vi "GUI_passive_Somatic_Test.vi"(0 "lang":string, 2 "Do test?":bool, 3 "Total trial":u16=80 min=1, 4 "Direction":i8=45) -> (7 "Direction 2":i8=20, 8 "stop 2":bool)   [LabVIEW 2012]
uses:
  <vilib>/Analysis/NI_AALBase.lvlib
  subVIs/Global_var.vi
  <vilib>/Utility/file.llb/Write To Spreadsheet File (DBL).vi
  <vilib>/Analysis/1siggen.llb/Riffle Array (I32).vi
panel:
  out "Response":u8
  out "Test Type":string
  out "Trial_index":u16
  out "Correct?":bool
  out "Response":path
  out "Trajectory":path
  out "Current Seq":u8
  out "Target":dbl[](array[numeric])
  out "flag":bool
  out "Directions":dbl[](array[numeric])
  out "Fz":dbl
  out "X":dbl
  out "Y":dbl
  out "Z":dbl
  out "Vx":dbl
  out "Vy":dbl
  out "Vz":dbl
  out "error out":errorcluster
  in  "Start?":bool
  out "Fx":dbl
  out "Fy":dbl
  out "Trial #":u16
  in  "stop":bool
  out "Canvas":picture
  # "Is the movement to the right or left of the body midline?"
  # "Delta robot kinetics information"
  # "degree"
types:
  T1 = typedef "Sound Output Task ID.ctl" = u32
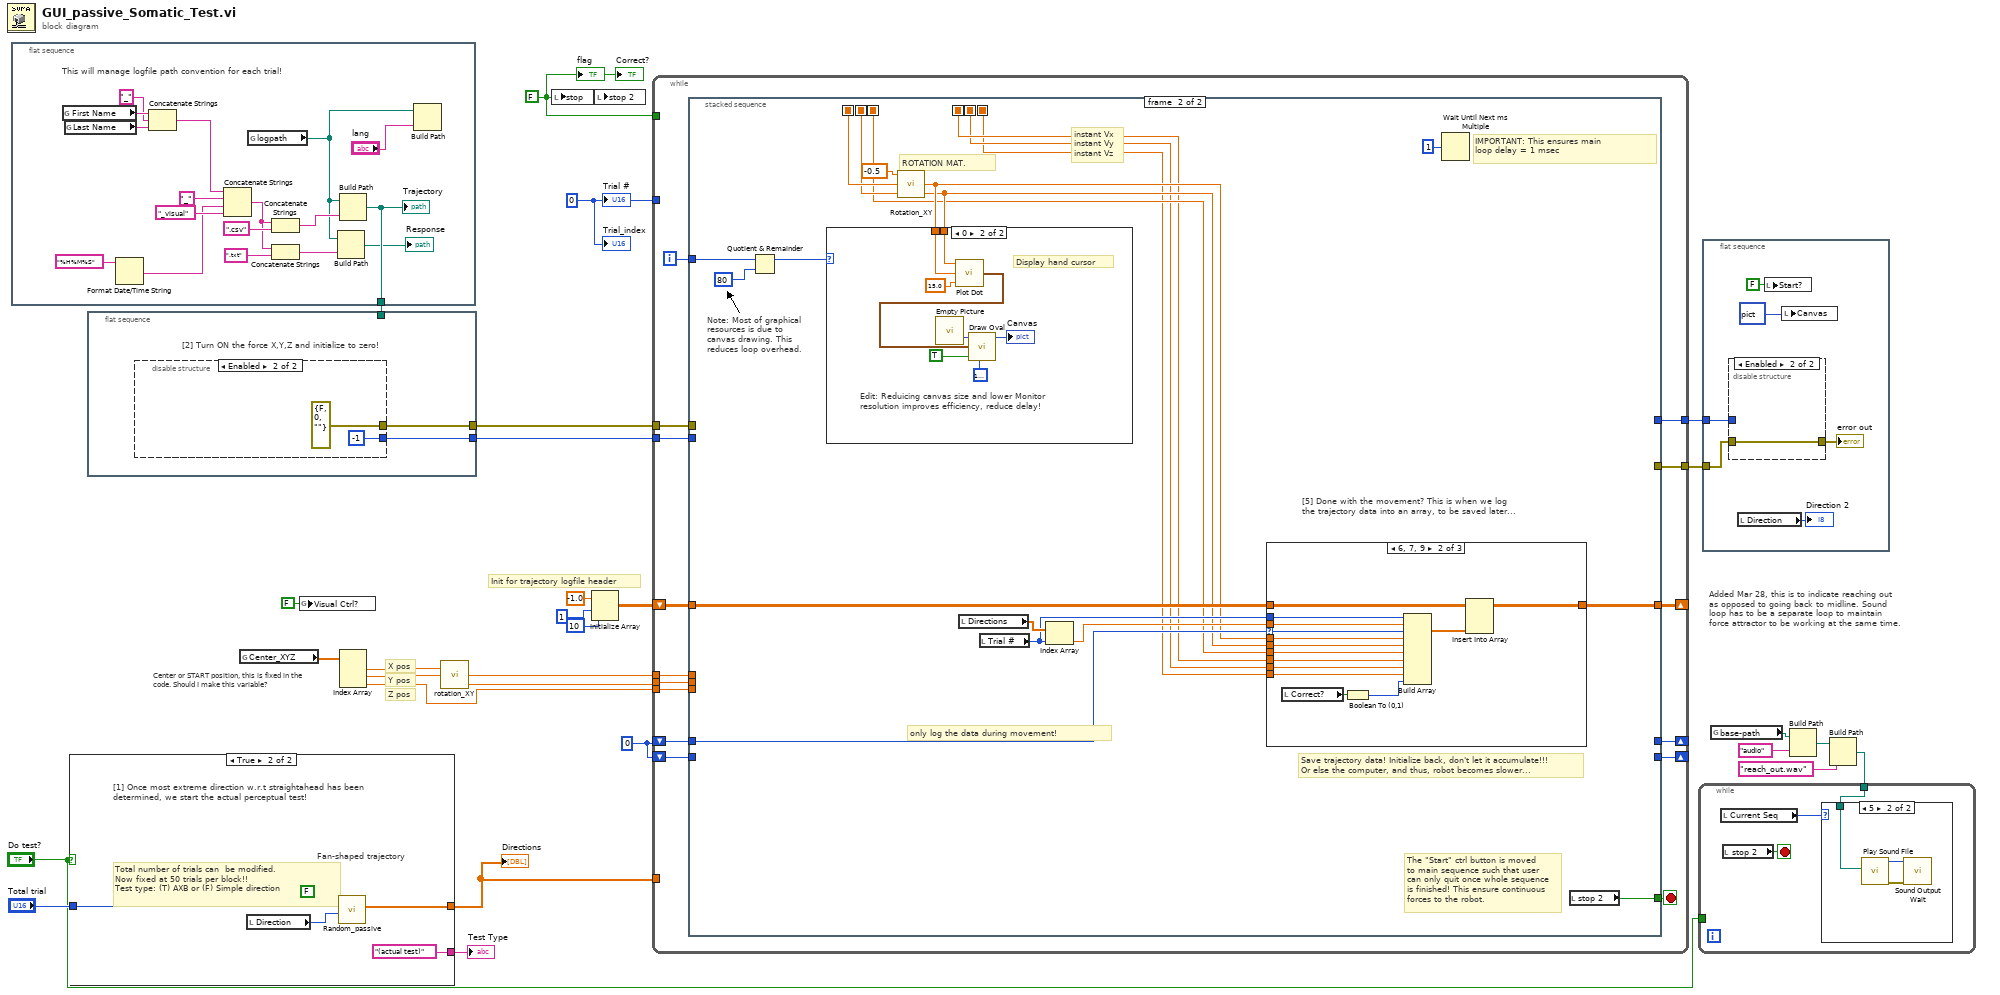
[diagram p0: block diagram]
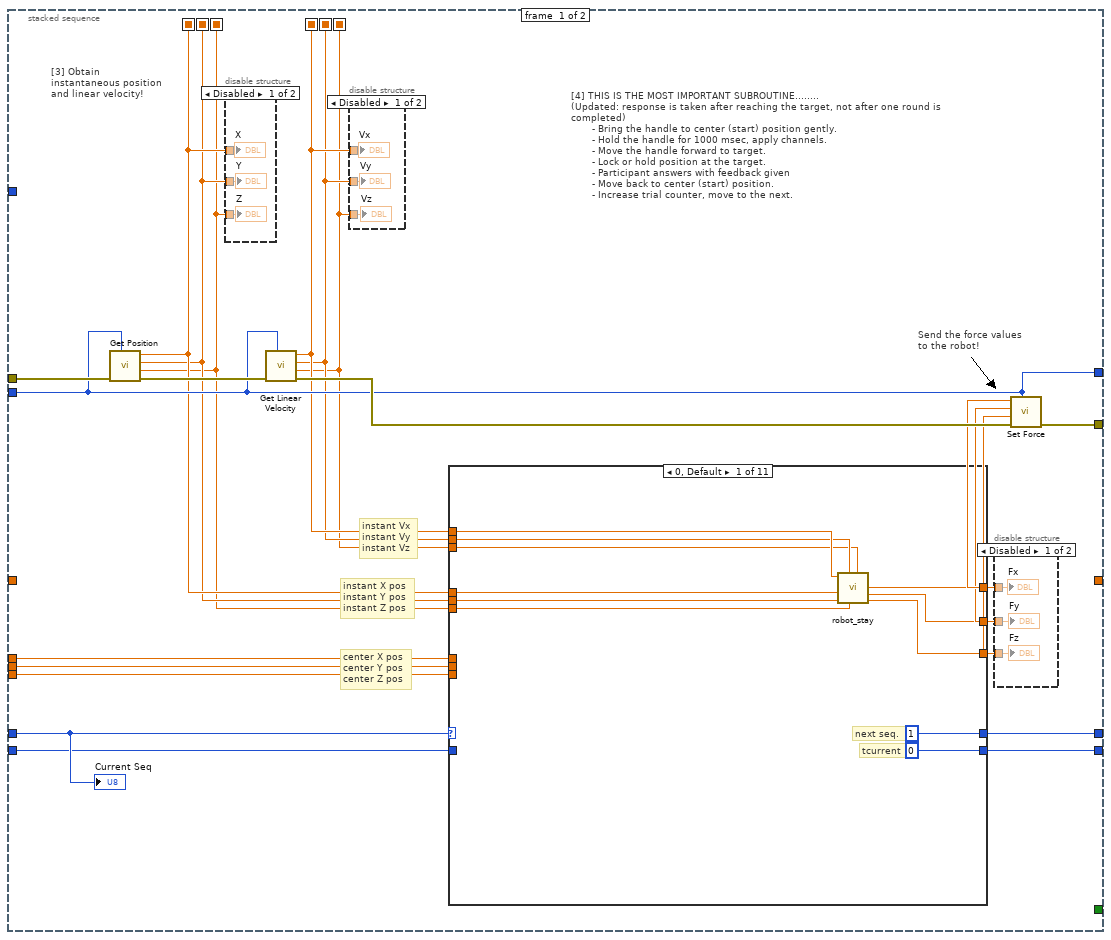
[diagram p3: hidden frame]
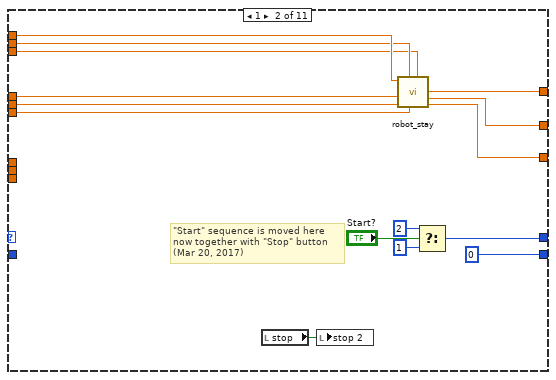
[diagram p7: hidden frame]
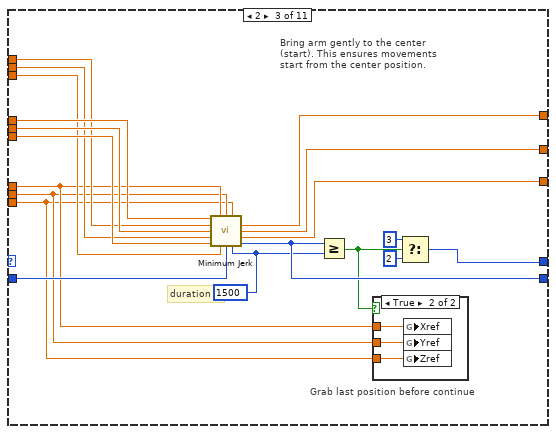
[diagram p8: hidden frame]
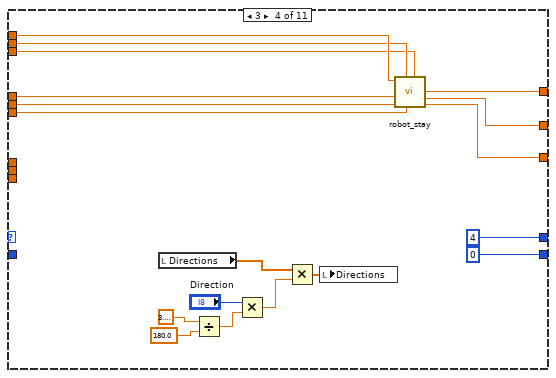
[diagram p10: hidden frame]
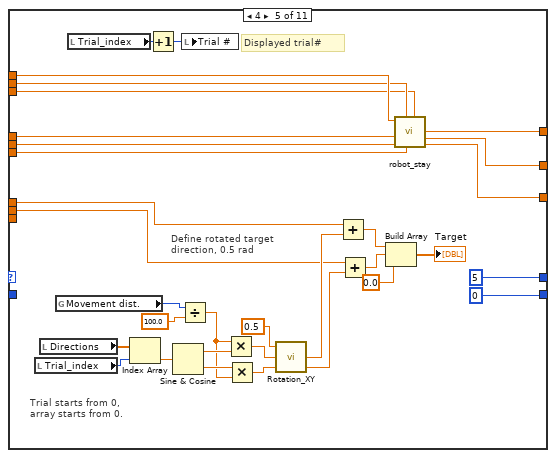
[diagram p11: hidden frame]
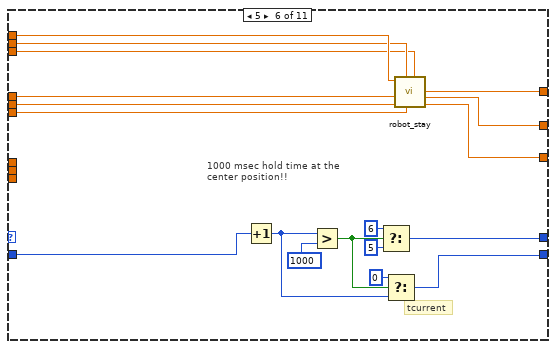
[diagram p12: hidden frame]
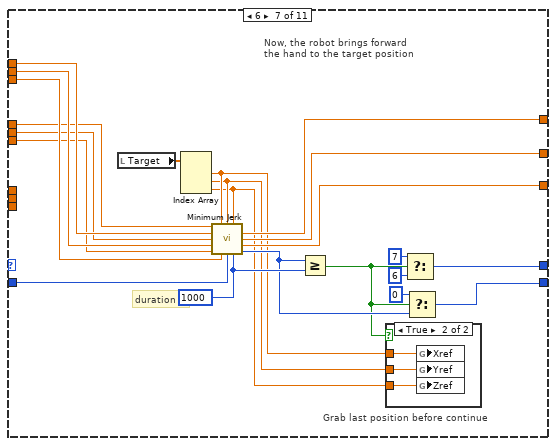
[diagram p13: hidden frame]
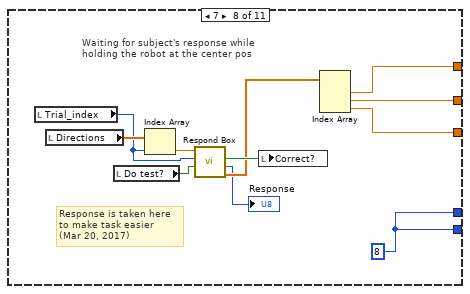
[diagram p15: hidden frame]
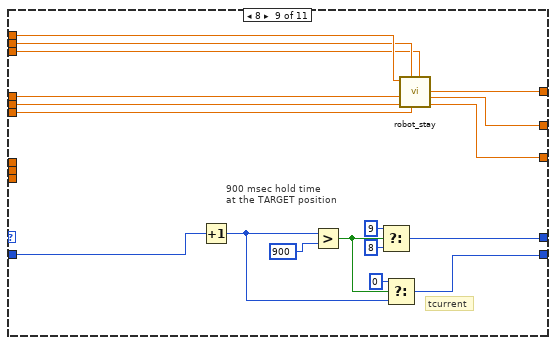
[diagram p16: hidden frame]
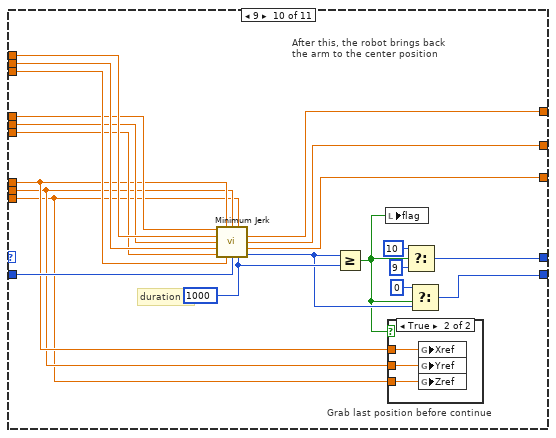
[diagram p17: hidden frame]
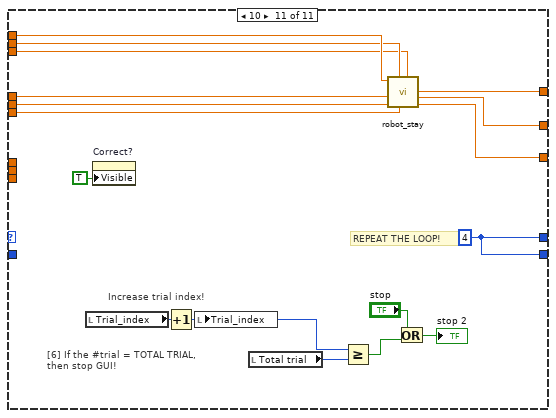
[diagram p19: hidden frame]
diagram:
  w16 = u16 0 ("y")
  w23 = FALSE ("stop")
  w25 = u16 0 ("ID")
  # "Added Mar 28, this is to indicate reaching out\nas opposed to going back to midline. Sound\nloop has to be a separate loop to maintain\nforce attractor to be working at the same time."
  # "Z pos"
  # "Y pos"
  # "X pos"
  # "Center or START position, this is fixed in the code. Should I make this variable?"
  # "Init for trajectory logfile header"
  n1 = flat-sequence {
    tunnel: [w31] -> w1
    frame #0 {
      # "This will manage logfile path convention for each trial!"
      n2 = global read "Global_var.vi" "First Name"() -> (w41:string)
      n3 = global read "Global_var.vi" "Last Name"() -> (w39:string)
      n4 = Format Date/Time String(time format string (%c)="%H%M%S") -> (date/time string=w43:string)  [unwired: 2 in]
      n5 = Concatenate Strings(w41, "_" ("string"), w39) -> (w38:string)
      n6 = Concatenate Strings(w38, "_" ("string"), w43, "_visual" ("string")) -> (w36:string)
      n7 = global read "Global_var.vi" "logpath"() -> (w33:path)
      n8 = Concatenate Strings(w36, ".csv" ("string")) -> (w34:string)
      n9 = Concatenate Strings(w36, ".txt" ("string")) -> (w32:string)
      n10 = Build Path(base path=w33, name or relative path=w32) -> (appended path=→"Response":path)
      n11 = Build Path(base path=w33, name or relative path=w34) -> (appended path=w31:path)
      "Trajectory" <- w31
      n12 = Build Path(base path=w33, name or relative path="lang") -> ()  [unwired: 1 out]
    }
  }
  n13 = case shown="True" "Do test?" {
    tunnel: [w46 w61] -> w12
    tunnel: "Total trial" -> [_ w60]
    tunnel: ["(extreme test) " "(actual test)"] -> w17
    frame False {
      # "[1] Determine min. perceivable direction, and randomise the presentation. (Darainy, 2017)."
      # "shuffle"
      n14 = local read "Total trial"() -> (w56:u16)
      n15 = Divide(x=w56, y=u8 2) -> (x/y=w55:dbl)
      n16 = Divide(x=w56, y=u8 2) -> (x/y=w50:dbl)
      n17 = Initialize Array(i8 1 ("element"), w55) -> (w49:i8[])
      n18 = Initialize Array(i8 -1 ("element"), w50) -> (w48:i8[])
      n19 = Build Array (concatenate)(w49, w48) -> (w47:i8[])
      n20 = call-poly <vilib>:"Riffle.vi"("X"=w47) -> ("Riffled {X}"=w46:i32[])  [unwired: 8 in, 2 out]
    }
    frame True {
      # "Fan-shaped trajectory"
      # "Total number of trials can  be modified.\nNow fixed at 50 trials per block!!\nTest type: (T) AXB or (F) Simple direction"
      # "[1] Once most extreme direction w.r.t straightahead has been determined, we start the actual perceptual test!"
      n21 = local read "Direction"() -> (w62:i8)
      n22 = call "Random_passive.vi"("Degree Max."=w62, "Total trial"=w60, "Test mode\n(Simple or AXB paradigm)?"=FALSE ("Test mode\n(Simple or AXB paradigm)?")) -> ("Target"=w61:dbl[])  [unwired: 5 in, 3 out]
    }
  }
  "Test Type" <- w17
  "Directions" <- w12
  n23 = flat-sequence {
    tunnel: [w64] -> w27
    tunnel: [w63] -> w26
    tunnel: w1 -> [_]
    frame #0 {
      # "[2] Turn ON the force X,Y,Z and initialize to zero!"
      n24 = disable-structure shown="Enabled" {
        disable-tunnel: [w66 errorcluster {"status"=FALSE, "code"=0, "source"=""} ("error out")] -> w64
        disable-tunnel: [w65 i8 -1 ("ID")] -> w63
        frame Disabled {
          w65 = i8 -1 ("ID")
          n25 = call <userlib>:"Open.vi"("error in (no error)"=errorcluster {"status"=FALSE, "code"=0, "source"=""} ("error out")) -> ("error out"=w67:errorcluster)  [unwired: 9 in, 1 out]
          n26 = call <userlib>:"Enable Force.vi"("error in (no error)"=w67, "ID"=w65, "val"=u8 1) -> ("error out"=w66:errorcluster)  [unwired: 7 in, 1 out]
        }
        frame Enabled {
        }
      }
    }
  }
  n27 = global read "Global_var.vi" "Center_XYZ"() -> (w13:dbl[])
  n28 = global write "Global_var.vi" "Visual Ctrl?"(FALSE ("Visual Ctrl?")) -> ()
  n29 = Index Array(array=w13) -> (element #1=w15:dbl, element #2=w14:dbl, element #3=w11:dbl)  [unwired: 3 in]
  n30 = call "rotation_XY.vi"("x_pos"=w14, "angle"=w15) -> ("rot_y"=w10:dbl, "rot_x"=w9:dbl)  [unwired: 2 in]
  n31 = local write "stop"(w23) -> ()
  n32 = Initialize Array(-1.0 ("vz out"), 1 ("dimension size"), 10 ("dimension size")) -> (w22:dbl[][])
  n33 = local write "stop 2"(w23) -> ()
  n34 = while {
    tunnel: w26 -> [w85]
    shift-right: [w86] -> _
    shift-left: w25 -> [w81]
    shift-right: [w83] -> _
    shift-left: w22 -> [w82]
    tunnel: [w79] -> w28
    tunnel: w16 -> [_]
    tunnel: w27 -> [w78]
    shift-right: [w76] -> _
    shift-left: w25 -> [w77]
    tunnel: w23 -> [_]
    tunnel: [w75] -> w24
    tunnel: w12 -> [_]
    tunnel: w9 -> [w74]
    tunnel: w10 -> [w73]
    tunnel: w11 -> [w72]
    i -> [w80]
    stop <- w84 stop-if-true
    n35 = stacked-sequence {
      seq-local: [w93 _] -> [_ w332]
      seq-local: [w90 _] -> [_ w329]
      seq-local: [w92 _] -> [_ w331]
      seq-local: [w91 _] -> [_ w330]
      seq-local: [w94 _] -> [_ w335]
      seq-local: [w95 _] -> [_ w336]
      tunnel: [w106 _] -> w86
      tunnel: w85 -> [w99 _]
      tunnel: [_ w328] -> w84
      tunnel: [_ w342] -> w83
      tunnel: w82 -> [_ w341]
      tunnel: w81 -> [w107 w338]
      tunnel: w80 -> [_ w346]
      tunnel: [w99 _] -> w79
      tunnel: w78 -> [w101 _]
      tunnel: w77 -> [w105 _]
      tunnel: [w104 _] -> w76
      tunnel: [w103 _] -> w75
      tunnel: w74 -> [w89 _]
      tunnel: w73 -> [w88 _]
      tunnel: w72 -> [w87 _]
      frame #0 {
        # "center X pos\ncenter Y pos\ncenter Z pos"
        # "[3] Obtain instantaneous position and linear velocity!"
        # "Send the force values to the robot!"
        # "instant Vx\ninstant Vy\ninstant Vz"
        # "[4] THIS IS THE MOST IMPORTANT SUBROUTINE........\n(Updated: response is taken after reaching the target, not after one round is completed)\n       - Bring the handle to center (start) position gently.\n       - Hold the handle for 1000 msec, apply channels.\n       - Move the handle forward to target.\n       - Lock or hold position at the target.\n       - Participant answers with feedback given\n       - Move back to center (start) position.\n       - Increase trial counter, move to the next."
        # "instant X pos\ninstant Y pos\ninstant Z pos"
        n36 = call <userlib>:"Get Position.vi"("ID"=w99, "error in (no error)"=w101) -> ("error out"=w102:errorcluster, "pz out"=w93:dbl, "py out"=w94:dbl, "px out"=w95:dbl)  [unwired: 5 in, 1 out]
        n37 = disable-structure shown="Disabled" {
          disable-tunnel: w95 -> [w113 _]
          disable-tunnel: w94 -> [w112 _]
          disable-tunnel: w93 -> [w111 _]
          frame Disabled {
            "Z" <- w111
            "Y" <- w112
            "X" <- w113
          }
          frame Enabled {
          }
        }
        n38 = call <userlib>:"Get Linear Velocity.vi"("ID"=w99, "error in (no error)"=w102) -> ("error out"=w100:errorcluster, "vz out"=w90:dbl, "vy out"=w91:dbl, "vx out"=w92:dbl)  [unwired: 5 in, 1 out]
        n39 = disable-structure shown="Disabled" {
          disable-tunnel: w92 -> [w116 _]
          disable-tunnel: w91 -> [w115 _]
          disable-tunnel: w90 -> [w114 _]
          frame Disabled {
            "Vz" <- w114
            "Vy" <- w115
            "Vx" <- w116
          }
          frame Enabled {
          }
        }
        n40 = case shown="0, Default" w107 {
          tunnel: [u8 1 ("ID") w128 w159 u8 4 ("ID") u8 5 ("ID") w232 w241 w268 w283 w294 w326] -> w106
          tunnel: [w122 w135 w155 w175 w185 w223 w244 w261 w271 w298 w322] -> w98
          tunnel: [w121 w134 w156 w174 w183 w222 w243 w263 w270 w297 w321] -> w97
          tunnel: w105 -> [_ _ w153 _ _ w230 w245 _ w279 w295 _]
          tunnel: [u16 0 ("tcurrent") u32 0 ("millisecond timer value") w158 u32 0 ("ID") u32 0 ("ID") w231 w239 w268 w281 w291 w326] -> w104
          tunnel: [w120 w133 w157 w173 w184 w221 w242 w262 w269 w296 w320] -> w96
          tunnel: w95 -> [w119 w138 w152 w178 w188 w226 w248 _ w274 w301 w325]
          tunnel: w94 -> [w118 w137 w151 w177 w187 w225 w247 _ w273 w300 w324]
          tunnel: w93 -> [w117 w136 w150 w176 w186 w224 w246 _ w272 w299 w323]
          tunnel: w92 -> [w125 w141 w149 w181 w191 w229 w251 _ w277 w304 w319]
          tunnel: w91 -> [w124 w140 w148 w180 w190 w228 w250 _ w276 w303 w318]
          tunnel: w90 -> [w123 w139 w147 w179 w189 w227 w249 _ w275 w302 w317]
          tunnel: w89 -> [_ _ w145 _ w197 _ _ _ _ w289 _]
          tunnel: w88 -> [_ _ w144 _ w196 _ _ _ _ w288 _]
          tunnel: w87 -> [_ _ w143 _ _ _ _ _ _ w287 _]
          frame 0, Default {
            # "next seq."
            # "tcurrent"
            n41 = call "robot_stay.vi"("Vz"=w123, "Z"=w117, "Vy"=w124, "Y"=w118, "X"=w119, "Vx"=w125) -> ("Fz"=w120:dbl, "Fy"=w121:dbl, "Fx"=w122:dbl)  [unwired: 3 in]
          }
          frame 1 {
            # "\"Start\" sequence is moved here \nnow together with \"Stop\" button\n(Mar 20, 2017)"
            n42 = local read "stop"() -> (w129:bool)
            n43 = local write "stop 2"(w129) -> ()
            n44 = call "robot_stay.vi"("Vz"=w139, "Z"=w136, "Vy"=w140, "Y"=w137, "X"=w138, "Vx"=w141) -> ("Fz"=w133:dbl, "Fy"=w134:dbl, "Fx"=w135:dbl)  [unwired: 3 in]
            n45 = Select(t=u8 2, s="Start?", f=u8 1) -> (s? t:f=w128:u8)
          }
          frame 2 {
            w154 = u16 1500 ("duration")
            # "Grab last position before continue"
            # "Bring arm gently to the center\n(start). This ensures movements\nstart from the center position."
            # "duration"
            n46 = call "Minimum Jerk.vi"("X"=w152, "Xfinal"=w145, "Yfinal"=w144, "Zfinal"=w143, "Vx"=w149, "Y"=w151, "Vy"=w148, "Z"=w150, "Vz"=w147, "current_n"=w153, "duration"=w154) -> ("Fx"=w155:dbl, "Fy"=w156:dbl, "Fz"=w157:dbl, "n out"=w158:u16)  [unwired: 1 out]
            n47 = Greater Or Equal?(x=w158, y=w154) -> (x >= y?=w146:bool)
            n48 = case shown="True" w146 {
              tunnel: w145 -> [_ w164]
              tunnel: w144 -> [_ w163]
              tunnel: w143 -> [_ w162]
              frame False {
              }
              frame True {
                n49 = global write "Global_var.vi" "Xref"(w164) -> ()
                n50 = global write "Global_var.vi" "Yref"(w163) -> ()
                n51 = global write "Global_var.vi" "Zref"(w162) -> ()
              }
            }
            n52 = Select(t=u8 3 ("ID"), s=w146, f=u8 2) -> (s? t:f=w159:u8)
          }
          frame 3 {
            n53 = local read "Directions"() -> (w166:dbl[])
            n54 = Divide(x=3.141592653589793, y=180.0) -> (x/y=w169:dbl)
            n55 = Multiply(x="Direction", y=w169) -> (x*y=w172:dbl)
            n56 = Multiply(x=w166, y=w172) -> (x*y=w167:dbl[])
            n57 = local write "Directions"(w167) -> ()
            n58 = call "robot_stay.vi"("Vz"=w179, "Z"=w176, "Vy"=w180, "Y"=w177, "X"=w178, "Vx"=w181) -> ("Fz"=w173:dbl, "Fy"=w174:dbl, "Fx"=w175:dbl)  [unwired: 3 in]
          }
          frame 4 {
            # "Displayed trial#"
            # "Trial starts from 0,\narray starts from 0."
            # "Define rotated target direction, 0.5 rad"
            n59 = local read "Trial_index"() -> (w210:u16)
            n60 = local read "Directions"() -> (w211:dbl[])
            n61 = global read "Global_var.vi" "Movement dist."() -> (w209:u8)
            n62 = local read "Trial_index"() -> (w192:u16)
            n63 = Index Array(array=w211, index=w210) -> (element=w212:dbl)
            n64 = Increment(x=w192) -> (x+1=w193:u16)
            n65 = Sine & Cosine(0:w212) -> (1:w213:dbl, 2:w214:dbl)
            n66 = Divide(x=w209, y=100.0) -> (x/y=w207:dbl)
            n67 = local write "Trial #"(w193) -> ()
            n68 = Multiply(x=w207, y=w213) -> (x*y=w205:dbl)
            n69 = Multiply(x=w214, y=w207) -> (x*y=w206:dbl)
            n70 = call "Rotation_XY.vi"("y_pos"=w206, "x_pos"=w205, "angle"=0.5 ("theta")) -> ("rot_y"=w202:dbl, "rot_x"=w203:dbl)  [unwired: 1 in]
            n71 = Add(x=w197, y=w203) -> (x+y=w200:dbl)
            n72 = Add(x=w196, y=w202) -> (x+y=w199:dbl)
            n73 = Build Array(w200, w199, 0.0 ("element")) -> (→"Target":dbl[])
            n74 = call "robot_stay.vi"("Vz"=w189, "Z"=w186, "Vy"=w190, "Y"=w187, "X"=w188, "Vx"=w191) -> ("Fz"=w184:dbl, "Fy"=w183:dbl, "Fx"=w185:dbl)  [unwired: 3 in]
          }
          frame 5 {
            # "1000 msec hold time at the center position!!"
            # "tcurrent"
            n75 = Increment(x=w230) -> (x+1=w215:u32)
            n76 = Greater?(x=w215, y=u32 1000) -> (0:w216:bool)
            n77 = Select(t=u8 6 ("ID"), s=w216, f=u8 5) -> (s? t:f=w232:u8)
            n78 = Select(t=u8 0 ("ID"), s=w216, f=w215) -> (s? t:f=w231:u32)
            n79 = call "robot_stay.vi"("Vz"=w227, "Z"=w224, "Vy"=w228, "Y"=w225, "X"=w226, "Vx"=w229) -> ("Fz"=w221:dbl, "Fy"=w222:dbl, "Fx"=w223:dbl)  [unwired: 3 in]
          }
          frame 6 {
            w252 = u16 1000 ("duration")
            # "Grab last position before continue"
            # "Now, the robot brings forward\nthe hand to the target position"
            # "duration"
            n80 = local read "Target"() -> (w237:dbl[])
            n81 = Index Array(array=w237) -> (element #1=w235:dbl, element #2=w234:dbl, element #3=w233:dbl)  [unwired: 3 in]
            n82 = call "Minimum Jerk.vi"("X"=w248, "Xfinal"=w235, "Yfinal"=w234, "Zfinal"=w233, "Vx"=w251, "Y"=w247, "Vy"=w250, "Z"=w246, "Vz"=w249, "current_n"=w245, "duration"=w252) -> ("Fx"=w244:dbl, "Fy"=w243:dbl, "Fz"=w242:dbl, "n out"=w238:u16)  [unwired: 1 out]
            n83 = Greater Or Equal?(x=w238, y=w252) -> (x >= y?=w236:bool)
            n84 = case shown="True" w236 {
              tunnel: w235 -> [_ w257]
              tunnel: w234 -> [_ w256]
              tunnel: w233 -> [_ w255]
              frame False {
              }
              frame True {
                n85 = global write "Global_var.vi" "Xref"(w257) -> ()
                n86 = global write "Global_var.vi" "Yref"(w256) -> ()
                n87 = global write "Global_var.vi" "Zref"(w255) -> ()
              }
            }
            n88 = Select(t=u8 7 ("ID"), s=w236, f=u8 6) -> (s? t:f=w241:u8)
            n89 = Select(t=u16 0, s=w236, f=w238) -> (s? t:f=w239:u16)
          }
          frame 7 {
            w268 = u8 8 ("ID")
            # "Response is taken here\nto make task easier\n(Mar 20, 2017)"
            # "Waiting for subject's response while\nholding the robot at the center pos"
            n90 = local read "Trial_index"() -> (w259:u16)
            n91 = local read "Directions"() -> (w267:dbl[])
            n92 = local read "Do test?"() -> (w260:bool)
            n93 = Index Array(array=w267, index=w259) -> (element=w266:dbl)
            n94 = call "Respond Box.vi"("Play?"=w260, "Trial#"=w259, "target"=w266) -> ("Force"=w264:dbl[], "out"=→"Response":i8, "Correct?"=w265:bool)  [unwired: 3 in]
            n95 = local write "Correct?"(w265) -> ()
            n96 = Index Array(array=w264) -> (element #1=w261:dbl, element #2=w263:dbl, element #3=w262:dbl)  [unwired: 3 in]
          }
          frame 8 {
            # "900 msec hold time\nat the TARGET position"
            # "tcurrent"
            n97 = Increment(x=w279) -> (x+1=w278:u32)
            n98 = Greater?(x=w278, y=u32 900) -> (0:w280:bool)
            n99 = Select(t=u8 9 ("ID"), s=w280, f=u8 8) -> (s? t:f=w283:u8)
            n100 = Select(t=u8 0 ("ID"), s=w280, f=w278) -> (s? t:f=w281:u32)
            n101 = call "robot_stay.vi"("Vz"=w275, "Z"=w272, "Vy"=w276, "Y"=w273, "X"=w274, "Vx"=w277) -> ("Fz"=w269:dbl, "Fy"=w270:dbl, "Fx"=w271:dbl)  [unwired: 3 in]
          }
          frame 9 {
            w305 = u16 1000 ("duration")
            # "Grab last position before continue"
            # "After this, the robot brings back\nthe arm to the center position"
            # "duration"
            n102 = call "Minimum Jerk.vi"("X"=w301, "Xfinal"=w289, "Yfinal"=w288, "Zfinal"=w287, "Vx"=w304, "Y"=w300, "Vy"=w303, "Z"=w299, "Vz"=w302, "current_n"=w295, "duration"=w305) -> ("Fx"=w298:dbl, "Fy"=w297:dbl, "Fz"=w296:dbl, "n out"=w292:u16)  [unwired: 1 out]
            n103 = Greater Or Equal?(x=w292, y=w305) -> (x >= y?=w290:bool)
            n104 = local write "flag"(w290) -> ()
            n105 = case shown="True" w290 {
              tunnel: w289 -> [_ w310]
              tunnel: w288 -> [_ w309]
              tunnel: w287 -> [_ w308]
              frame False {
              }
              frame True {
                n106 = global write "Global_var.vi" "Xref"(w310) -> ()
                n107 = global write "Global_var.vi" "Yref"(w309) -> ()
                n108 = global write "Global_var.vi" "Zref"(w308) -> ()
              }
            }
            n109 = Select(t=u8 10 ("ID"), s=w290, f=u8 9) -> (s? t:f=w294:u8)
            n110 = Select(t=u16 0, s=w290, f=w292) -> (s? t:f=w291:u16)
          }
          frame 10 {
            w326 = u8 4 ("ID")
            # "REPEAT THE LOOP!"
            # "[6] If the #trial = TOTAL TRIAL, \nthen stop GUI!"
            # "Increase trial index!"
            n111 = local read "Trial_index"() -> (w316:u16)
            n112 = property on="Correct?" class="Bool (strict)"("Visible"=TRUE ("stop")) -> ()  [unwired: 2 in, 2 out]
            n113 = Increment(x=w316) -> (x+1=w314:u16)
            n114 = local write "Trial_index"(w314) -> ()
            n115 = local read "Total trial"() -> (w315:u16)
            n116 = Greater Or Equal?(x=w314, y=w315) -> (x >= y?=w311:bool)
            n117 = call "robot_stay.vi"("Vz"=w317, "Z"=w323, "Vy"=w318, "Y"=w324, "X"=w325, "Vx"=w319) -> ("Fz"=w320:dbl, "Fy"=w321:dbl, "Fx"=w322:dbl)  [unwired: 3 in]
            n118 = Or(x="stop", y=w311) -> (x .or. y?=→"stop 2":bool)
          }
        }
        n119 = disable-structure shown="Disabled" {
          disable-tunnel: w98 -> [w110 _]
          disable-tunnel: w97 -> [w109 _]
          disable-tunnel: w96 -> [w108 _]
          frame Disabled {
            "Fy" <- w109
            "Fx" <- w110
            "Fz" <- w108
          }
          frame Enabled {
          }
        }
        n120 = call <userlib>:"Set Force.vi"("ID"=w99, "error in (no error)"=w100, "fz"=w96, "fy"=w97, "fx"=w98) -> ("error out"=w103:errorcluster)  [unwired: 5 in, 1 out]
        "Current Seq" <- w107
      }
      frame #1 {
        # "Save trajectory data! Initialize back, don't let it accumulate!!!\nOr else the computer, and thus, robot becomes slower..."
        # "The \"Start\" ctrl button is moved\nto main sequence such that user\ncan only quit once whole sequence\nis finished! This ensure continuous\nforces to the robot."
        # "instant Vx\ninstant Vy\ninstant Vz"
        # "Note: Most of graphical resources is due to canvas drawing. This\nreduces loop overhead."
        # "IMPORTANT: This ensures main \nloop delay = 1 msec"
        # "ROTATION MAT."
        # "only log the data during movement!"
        # "[5] Done with the movement? This is when we log\nthe trajectory data into an array, to be saved later..."
        n121 = Quotient & Remainder(x=w346, y=80) -> (x-y*floor(x/y)=w339:i32)  [unwired: 1 out]
        n122 = call "Rotation_XY.vi"("y_pos"=w335, "x_pos"=w336, "angle"=-0.5 ("theta")) -> ("rot_y"=w333:dbl, "rot_x"=w334:dbl)  [unwired: 1 in]
        n123 = case shown="0" w339 {
          tunnel: w334 -> [_ w381]
          tunnel: w333 -> [_ w382]
          frame 1, Default {
            # "I disable the visual cues"
          }
          frame 0 {
            # "Edit: Reduicing canvas size and lower Monitor resolution improves efficiency, reduce delay!"
            # "Display hand cursor"
            n124 = call "Empty Picture"() -> ("empty picture"=w380:picture)
            n125 = call "Plot Dot.vi"("Diameter"=15.0 ("Size"), "Y"=w381, "X"=w382) -> ("Cluster"=w379:cluster{dbl, dbl, dbl, dbl})
            n126 = call <vilib>:"Draw Oval.vi"("picture"=w380, "rect"=w379, "fill?(F)"=TRUE, "color(black)"=u32 16777226) -> ("new picture"=→"Canvas":picture)  [unwired: 5 in]
          }
        }
        n127 = local read "Directions"() -> (w344:dbl[])
        n128 = local read "Trial #"() -> (w343:u16)
        n129 = Index Array(array=w344, index=w343) -> (element=w345:dbl)
        n130 = case shown="6, 7, 9" w338 {
          selector: w338 -> [_ w357 _]
          tunnel: [w348 w361 dbl[][] []] -> w342
          tunnel: w341 -> [w348 w360 w375]
          tunnel: w345 -> [_ w359 w366]
          tunnel: w343 -> [_ w358 w367]
          tunnel: w334 -> [_ w355 _]
          tunnel: w333 -> [_ w354 _]
          tunnel: w332 -> [_ w353 _]
          tunnel: w331 -> [_ w351 _]
          tunnel: w330 -> [_ w350 _]
          tunnel: w329 -> [_ w349 _]
          frame 0, Default {
          }
          frame 6, 7, 9 {
            n131 = local read "Correct?"() -> (w356:bool)
            n132 = Boolean To (0,1)(Boolean=w356) -> (0, 1=w352:i16)
            n133 = Build Array(w358, w359, w357, w355, w354, w353, w351, w350, w349, w352) -> (w362:dbl[])
            n134 = Insert Into Array(array=w360, new element=w362) -> (w361:dbl[][])  [unwired: 2 in]
          }
          frame 10 {
            n135 = local read "Trajectory"() -> (w378:path)
            n136 = local read "Response"() -> (w364:u8)
            n137 = local read "Correct?"() -> (w368:bool)
            n138 = Boolean To (0,1)(Boolean=w368) -> (0, 1=w363:i16)
            n139 = call-poly <vilib>:"Write To Spreadsheet File.vi"("delimiter (\\t)"="," ("delimiter (\\t)"), "format (%.3f)"="%.6f", "append to file? (new file:F)"=TRUE, "2D data"=w375, "file path (dialog if empty)"=w378) -> ()  [unwired: 3 in, 1 out]
            n140 = Build Array(w367, w366, w364, w363) -> (w365:dbl[])
            n141 = local read "Response"() -> (w369:path)
            n142 = call-poly <vilib>:"Write To Spreadsheet File.vi"("delimiter (\\t)"="," ("delimiter (\\t)"), "format (%.3f)"="%.6f", "append to file? (new file:F)"=TRUE, "1D data"=w365, "file path (dialog if empty)"=w369) -> ()  [unwired: 3 in, 1 out]
          }
        }
        n143 = Wait Until Next ms Multiple(millisecond multiple=u32 1) -> ()  [unwired: 1 out]
        n144 = local read "stop 2"() -> (w328:bool)
      }
    }
  }
  n145 = flat-sequence {
    tunnel: w28 -> [w392]
    tunnel: w24 -> [w388]
    frame #0 {
      n146 = disable-structure shown="Enabled" {
        disable-tunnel: w392 -> [w395 _]
        disable-tunnel: w388 -> [w394 w396]
        disable-tunnel: [w393 w396] -> w387
        frame Disabled {
          # "Close!"
          n147 = call <userlib>:"Close.vi"("error in (no error)"=w394, "ID"=w395) -> ("error out"=w393:errorcluster)  [unwired: 8 in, 1 out]
        }
        frame Enabled {
        }
      }
      "error out" <- w387
      n148 = local read "Direction"() -> (→"Direction 2":i8)
      n149 = local write "Start?"(FALSE ("start")) -> ()
      n150 = local write "Canvas"(picture data[5B] ("Canvas")) -> ()
    }
  }
  n151 = global read "Global_var.vi" "base-path"() -> (w5:path)
  n152 = Build Path(base path=w5, name or relative path="audio") -> (appended path=w2:path)
  n153 = Build Path(base path=w2, name or relative path="reach_out.wav") -> (appended path=w3:path)
  n154 = while {
    tunnel: w3 -> [w398]
    tunnel: "Do test?" -> [_]
    stop <- w397 stop-if-true
    n155 = local read "Current Seq"() -> (w399:u8)
    n156 = local read "stop 2"() -> (w397:bool)
    n157 = case shown="5" w399 {
      tunnel: w398 -> [_ w400]
      frame 0, Default {
      }
      frame 5 {
        n158 = call <vilib>:"Play Sound File.vi"("path"=w400) -> ("error out"=w402:errorcluster, "task ID"=w401:T1)  [unwired: 9 in]
        n159 = call <vilib>:"Sound Output Wait.vi"("error in (no error)"=w402, "task ID"=w401) -> ()  [unwired: 8 in, 2 out]
      }
    }
  }
  "flag" <- w23
  "Trial #" <- w16
  "Correct?" <- w23
  "Trial_index" <- w16
